vi "Left Button.vi"(7 "Index In in":i32, 8 "error in (no error)":errorcluster, 9 "Data In":T1, 10 "Button Index":i32, 11 "Button in":refnum<class "Button.lvclass">) -> (0 "error out":errorcluster, 1 "Data out":T1, 2 "Data Changed ?":bool, 3 "Button out":refnum<class "Button.lvclass">, 5 "Index In out":i32)   [LabVIEW 2012, in "Button.lvclass"]
uses:
  Button.lvclass
  Toolbar Data.ctl
  Type Defs/Button Events.ctl
  Type Defs/Button Status.ctl
  Toolbar.xctl
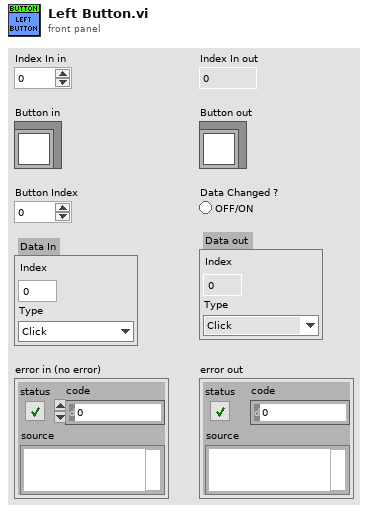
[diagram p1: front panel]
types:
  T1 = typedef "Toolbar.xctl/Toolbar Data.ctl" = cluster{"Index":i32, "Type":T2}
  T2 = typedef "Button.lvclass/Button Events.ctl" = enum16{"Click", "Latch", "Unlatch"}
  T3 = typedef "Button.lvclass/Button Status.ctl" = enum16{"Off", "Hover", "On", "Disabled"}
  T4 = typedef "Button.lvclass/Button Type.ctl" = enum16{"Transitory", "Latching"}
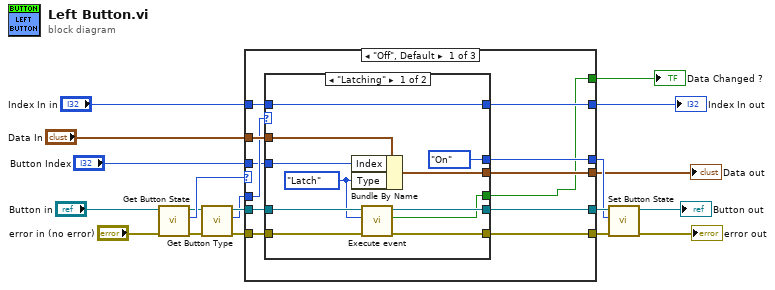
[diagram p0: block diagram]
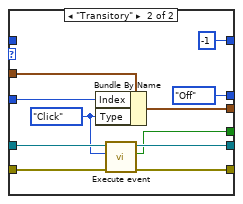
[diagram p2: hidden frame]
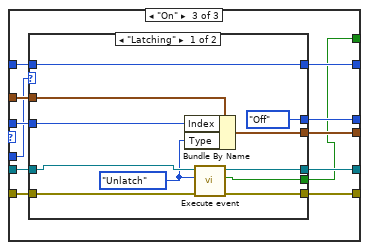
[diagram p4: hidden frame]
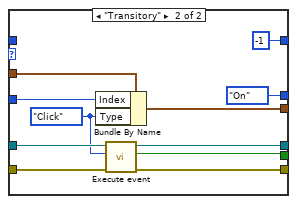
[diagram p5: hidden frame]
diagram:
  n1 = call-dynamic "Get Button State.vi"("error in (no error)"="error in (no error)", "Button in"="Button in") -> ("error out"=w12:errorcluster, "State"=w8:T3, "Button out"=w7:refnum<class "Button.lvclass">)  [unwired: 7 out]
  n2 = call-dynamic "Get Button Type.vi"("error in (no error)"=w12, "Button in"=w7) -> ("error out"=w14:errorcluster, "Type"=w9:T4, "Button out"=w10:refnum<class "Button.lvclass">)  [unwired: 7 out]
  n3 = case shown="\"Off\", Default" w8 {
    selector: w8 -> [_ w58 _]
    tunnel: [w23 w58 w62] -> w6
    tunnel: [w31 w57 w68] -> w5
    tunnel: "Data In" -> [w30 w57 w70]
    tunnel: "Button Index" -> [w28 _ w69]
    tunnel: [w20 _ w59] -> w4
    tunnel: w9 -> [w29 _ w67]
    tunnel: w10 -> [w27 w56 w66]
    tunnel: [w26 w56 w65] -> w11
    tunnel: [w24 w55 w64] -> w13
    tunnel: w14 -> [w25 w55 w63]
    tunnel: [w21 w54 w60] -> w18
    tunnel: "Index In in" -> [w22 w54 w61]
    frame "Off", Default {
      n4 = case shown="\"Latching\"" w29 {
        tunnel: w30 -> [w42 w53]
        tunnel: [w41 w52] -> w31
        tunnel: w28 -> [w40 w51]
        tunnel: w27 -> [w39 w50]
        tunnel: [w38 w49] -> w26
        tunnel: w25 -> [w36 w47]
        tunnel: [w35 w46] -> w24
        tunnel: [Button_Status."On" ("t") Button_Status."Off" ("t")] -> w23
        tunnel: [w33 -1 ("Index In")] -> w21
        tunnel: w22 -> [w33 _]
        tunnel: [w32 w43] -> w20
        frame "Latching" {
          w37 = Button_Events."Latch" ("Type")
          n5 = Bundle By Name(cluster=w42, "Index"=w40, "Type"=w37) -> (w41:T1)
          n6 = call-dynamic "Execute event.vi"("error in (no error)"=w36, "Button Event"=w37, "Button in"=w39) -> ("error out"=w35:errorcluster, "Value Changed ?"=w32:bool, "Button out"=w38:refnum<class "Button.lvclass">)  [unwired: 1 in, 5 out]
        }
        frame "Transitory" {
          w48 = Button_Events."Click" ("Type")
          n7 = Bundle By Name(cluster=w53, "Index"=w51, "Type"=w48) -> (w52:T1)
          n8 = call-dynamic "Execute event.vi"("error in (no error)"=w47, "Button Event"=w48, "Button in"=w50) -> ("error out"=w46:errorcluster, "Value Changed ?"=w43:bool, "Button out"=w49:refnum<class "Button.lvclass">)  [unwired: 1 in, 5 out]
        }
      }
    }
    frame "Disabled" {
    }
    frame "On" {
      n9 = case shown="\"Latching\"" w67 {
        tunnel: w70 -> [w81 w92]
        tunnel: [w80 w91] -> w68
        tunnel: w69 -> [w79 w90]
        tunnel: w66 -> [w78 w89]
        tunnel: [w77 w87] -> w65
        tunnel: w63 -> [w75 w85]
        tunnel: [w74 w86] -> w64
        tunnel: [Button_Status."Off" ("State") Button_Status."On" ("State")] -> w62
        tunnel: [w72 -1 ("Index In")] -> w60
        tunnel: w61 -> [w72 _]
        tunnel: [w71 w82] -> w59
        frame "Latching" {
          w76 = Button_Events."Unlatch" ("Type")
          n10 = Bundle By Name(cluster=w81, "Index"=w79, "Type"=w76) -> (w80:T1)
          n11 = call-dynamic "Execute event.vi"("error in (no error)"=w75, "Button Event"=w76, "Button in"=w78) -> ("error out"=w74:errorcluster, "Value Changed ?"=w71:bool, "Button out"=w77:refnum<class "Button.lvclass">)  [unwired: 1 in, 5 out]
        }
        frame "Transitory" {
          w88 = Button_Events."Click" ("Type")
          n12 = Bundle By Name(cluster=w92, "Index"=w90, "Type"=w88) -> (w91:T1)
          n13 = call-dynamic "Execute event.vi"("error in (no error)"=w85, "Button Event"=w88, "Button in"=w89) -> ("error out"=w86:errorcluster, "Value Changed ?"=w82:bool, "Button out"=w87:refnum<class "Button.lvclass">)  [unwired: 1 in, 5 out]
        }
      }
    }
  }
  "Index In out" <- w18
  "Data out" <- w5
  "Data Changed ?" <- w4
  n14 = call-dynamic "Set Button State.vi"("error in (no error)"=w13, "State"=w6, "Button in"=w11) -> ("error out"=→"error out":errorcluster, "Button out"=→"Button out":refnum<class "Button.lvclass">)  [unwired: 7 out]
